vi "Create All Message Queues.vi"(8 "error in (no error)":errorcluster) -> (0 "error out":errorcluster, 3 "Message Queues out":T1)   [LabVIEW 2023, in "Tenney Message Queue.lvlib"]
doc: "This VI creates and initializes all the message queues for your application. If your application requires more than one message queue, right-click the \"Message Queues\" constant above and select Open Type Def. Add the new Message Queue(s) to the type definition, then initialize them in this VI."
uses:
  Tenney Message Queue.lvlib
  All Message Queues.ctl
  Message Cluster.ctl
  Enqueue Message (Single).vi
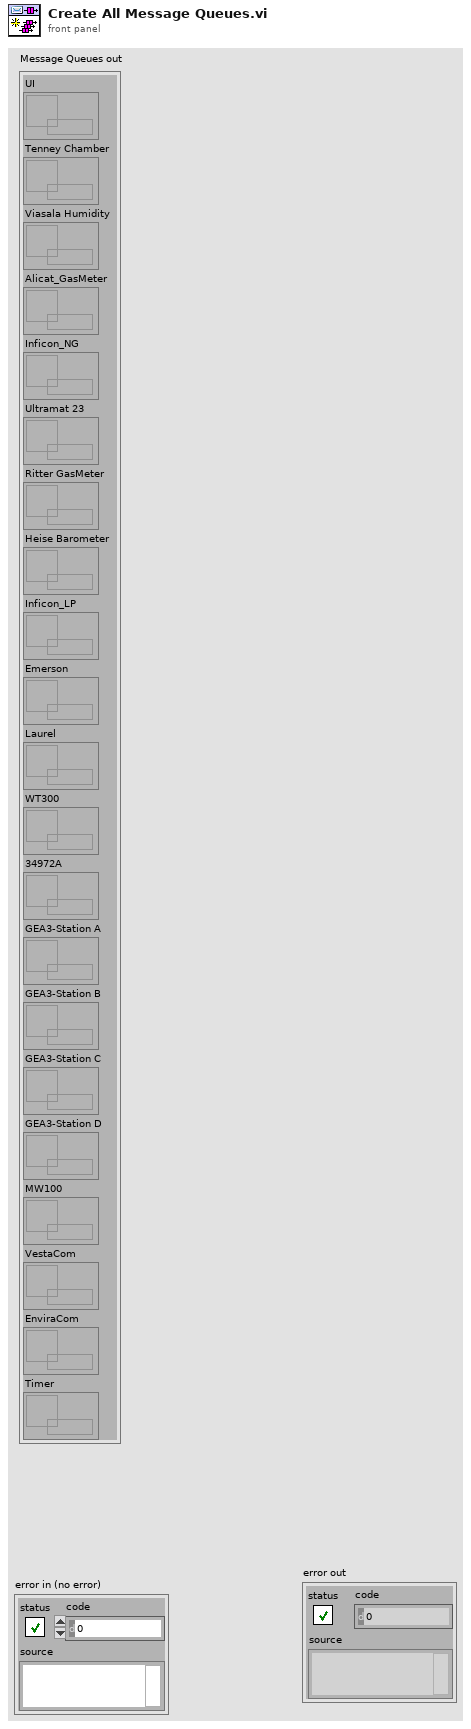
[diagram p1: front panel]
types:
  T1 = typedef "Tenney Message Queue.lvlib/All Message Queues.ctl" = cluster{"UI":refnum<queue>, "Tenney Chamber":refnum<queue>, "Viasala Humidity":refnum<queue>, "Alicat_GasMeter":refnum<queue>, "Inficon_NG":refnum<queue>, "Ultramat 23":refnum<queue>, "Ritter GasMeter":refnum<queue>, "Heise Barometer":refnum<queue>, "Inficon_LP":refnum<queue>, "Emerson":refnum<queue>, "Laurel":refnum<queue>, "WT300":refnum<queue>, "34972A":refnum<queue>, "GEA3-Station A":refnum<queue>, "GEA3-Station B":refnum<queue>, "GEA3-Station C":refnum<queue>, "GEA3-Station D":refnum<queue>, "MW100":refnum<queue>, "VestaCom":refnum<queue>, "EnviraCom":refnum<queue>, "Timer":refnum<queue>}
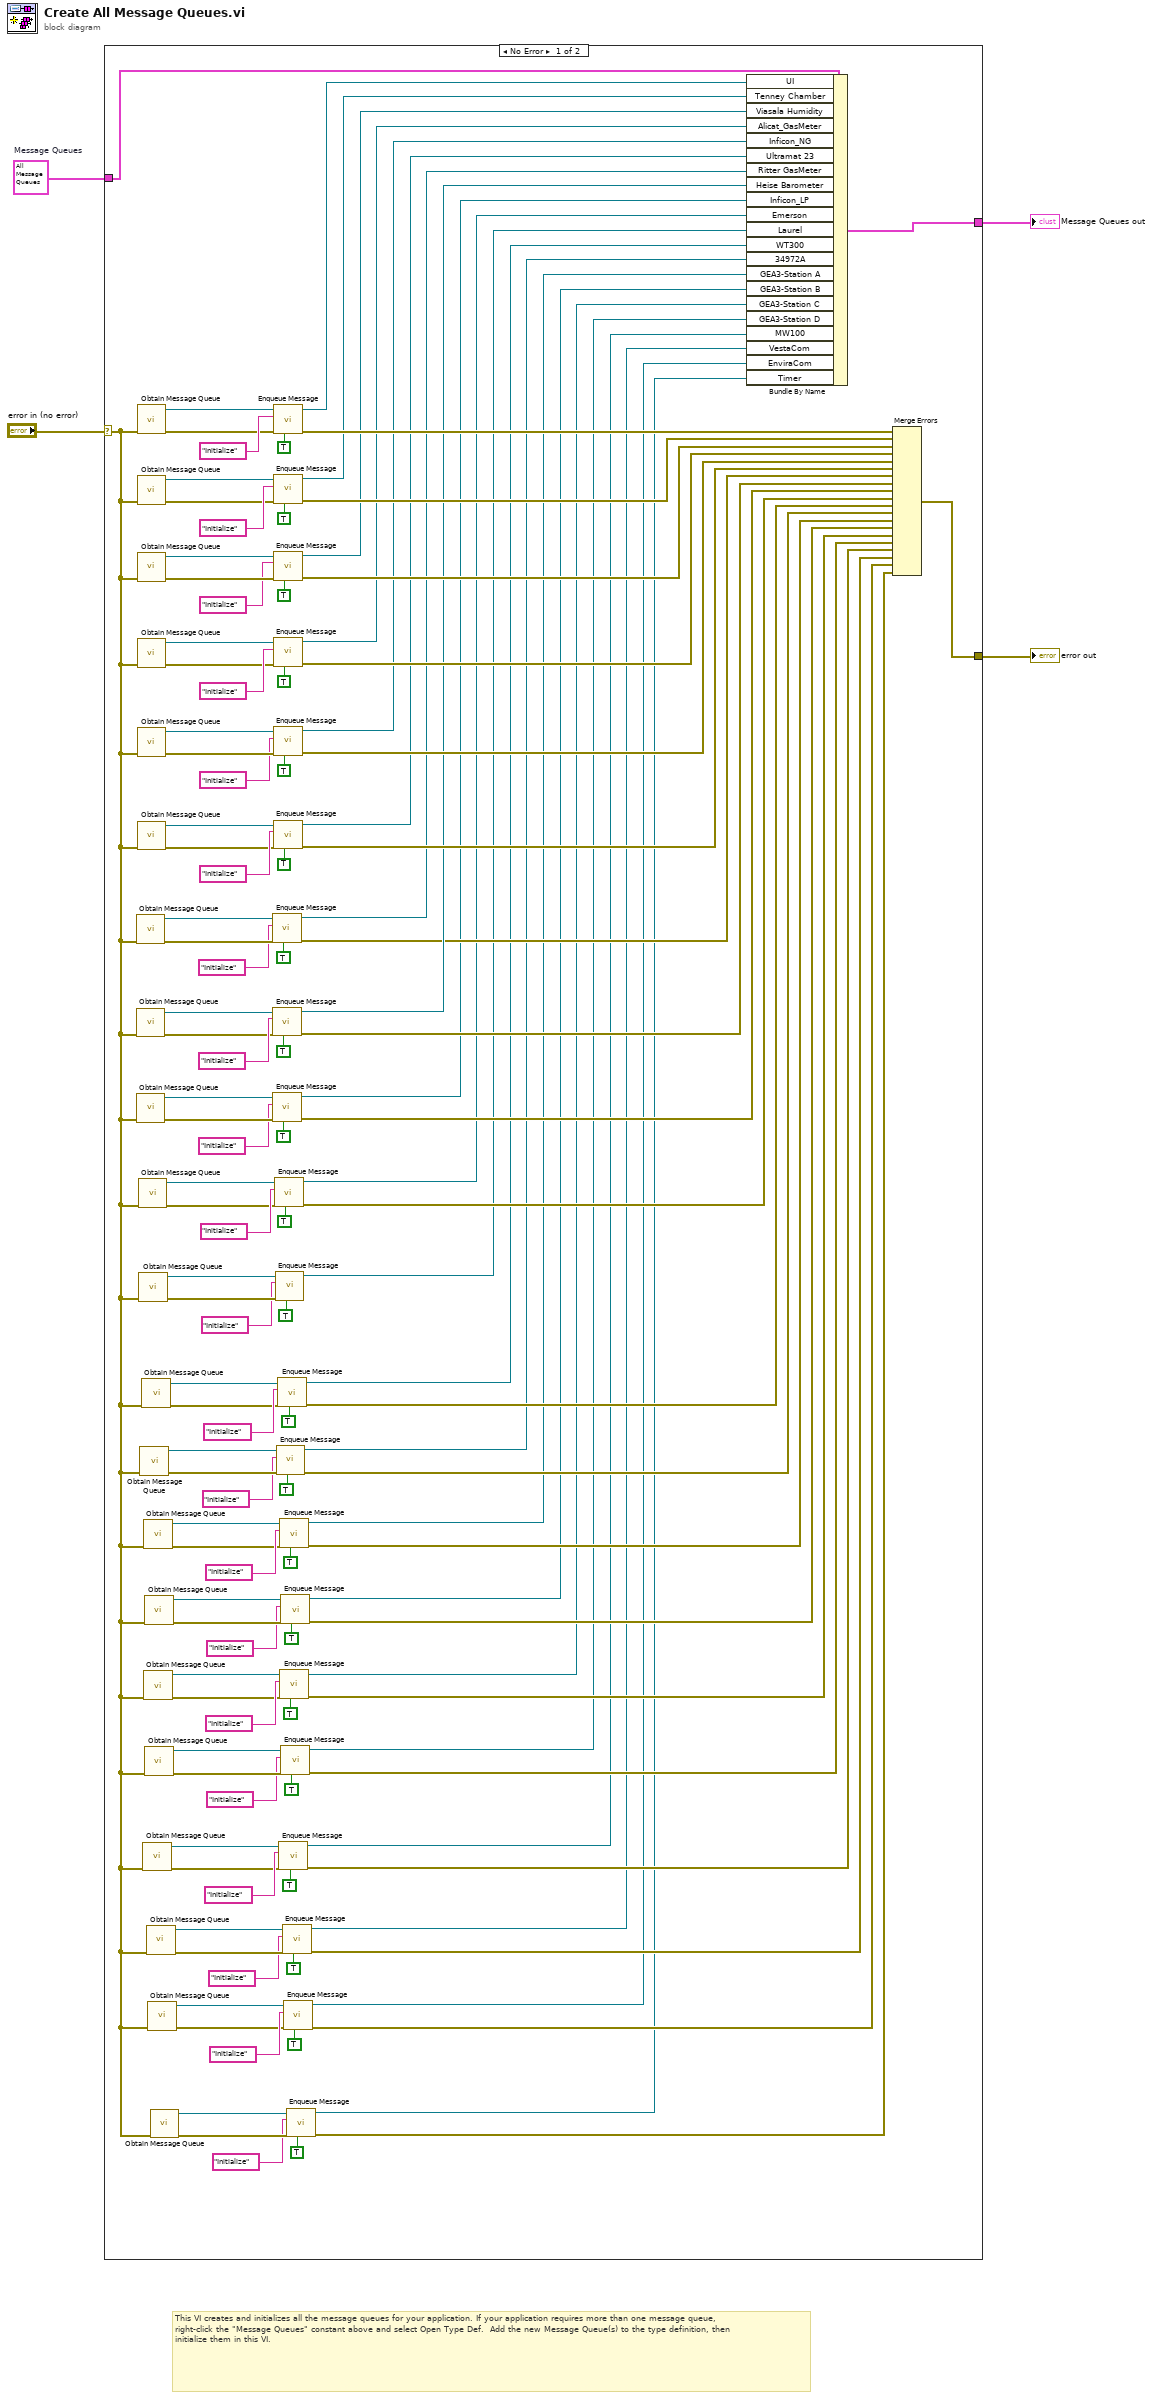
[diagram p0: block diagram]
diagram:
  w1 = T1 {"UI"=refnum, "Tenney Chamber"=refnum, "Viasala Humidity"=refnum, "Alicat_GasMeter"=refnum, "Inficon_NG"=refnum, "Ultramat 23"=refnum, "Ritter GasMeter"=refnum, "Heise Barometer"=refnum, "Inficon_LP"=refnum, "Emerson"=refnum, "Laurel"=refnum, "WT300"=refnum, "34972A"=refnum, "GEA3-Station A"=refnum, "GEA3-Station B"=refnum, "GEA3-Station C"=refnum, "GEA3-Station D"=refnum, "MW100"=refnum, "VestaCom"=refnum, "EnviraCom"=refnum, "Timer"=refnum}  # Message Queues
  # "This VI creates and initializes all the message queues for your application. If your application requires more than one message queue, right-click the \"Message Queues\" constant above and select Open Type Def.  Add the new Message Queue(s) to the type definition, then initialize them in this VI."
  n1 = case shown="No Error" "error in (no error)" {
    selector: "error in (no error)" -> [w7 w135]
    tunnel: [w127 w135] -> w4
    tunnel: [w133 w134] -> w3
    tunnel: w1 -> [w126 w134]
    frame No Error {
      n2 = call "Obtain Message Queue.vi"("error in (no error)"=w7) -> ("error out"=w94:errorcluster, "Message Queue"=w93:refnum<queue>)  [unwired: 9 in]
      n3 = call "Obtain Message Queue.vi"("error in (no error)"=w7) -> ("error out"=w87:errorcluster, "Message Queue"=w88:refnum<queue>)  [unwired: 9 in]
      n4 = call "Obtain Message Queue.vi"("error in (no error)"=w7) -> ("error out"=w82:errorcluster, "Message Queue"=w81:refnum<queue>)  [unwired: 9 in]
      n5 = call "Obtain Message Queue.vi"("error in (no error)"=w7) -> ("error out"=w130:errorcluster, "Message Queue"=w131:refnum<queue>)  [unwired: 9 in]
      n6 = call "Obtain Message Queue.vi"("error in (no error)"=w7) -> ("error out"=w119:errorcluster, "Message Queue"=w120:refnum<queue>)  [unwired: 9 in]
      n7 = call "Obtain Message Queue.vi"("error in (no error)"=w7) -> ("error out"=w118:errorcluster, "Message Queue"=w117:refnum<queue>)  [unwired: 9 in]
      n8 = call "Obtain Message Queue.vi"("error in (no error)"=w7) -> ("error out"=w109:errorcluster, "Message Queue"=w110:refnum<queue>)  [unwired: 9 in]
      n9 = call "Obtain Message Queue.vi"("error in (no error)"=w7) -> ("error out"=w106:errorcluster, "Message Queue"=w105:refnum<queue>)  [unwired: 9 in]
      n10 = call "Obtain Message Queue.vi"("error in (no error)"=w7) -> ("error out"=w97:errorcluster, "Message Queue"=w98:refnum<queue>)  [unwired: 9 in]
      n11 = call "Obtain Message Queue.vi"("error in (no error)"=w7) -> ("error out"=w73:errorcluster, "Message Queue"=w74:refnum<queue>)  [unwired: 9 in]
      n12 = call "Obtain Message Queue.vi"("error in (no error)"=w7) -> ("error out"=w70:errorcluster, "Message Queue"=w69:refnum<queue>)  [unwired: 9 in]
      n13 = call "Obtain Message Queue.vi"("error in (no error)"=w7) -> ("error out"=w59:errorcluster, "Message Queue"=w58:refnum<queue>)  [unwired: 9 in]
      n14 = call "Obtain Message Queue.vi"("error in (no error)"=w7) -> ("error out"=w62:errorcluster, "Message Queue"=w63:refnum<queue>)  [unwired: 9 in]
      n15 = call "Obtain Message Queue.vi"("error in (no error)"=w7) -> ("error out"=w26:errorcluster, "Message Queue"=w27:refnum<queue>)  [unwired: 9 in]
      n16 = call "Obtain Message Queue.vi"("error in (no error)"=w7) -> ("error out"=w50:errorcluster, "Message Queue"=w51:refnum<queue>)  [unwired: 9 in]
      n17 = call "Obtain Message Queue.vi"("error in (no error)"=w7) -> ("error out"=w42:errorcluster, "Message Queue"=w43:refnum<queue>)  [unwired: 9 in]
      n18 = call "Obtain Message Queue.vi"("error in (no error)"=w7) -> ("error out"=w49:errorcluster, "Message Queue"=w48:refnum<queue>)  [unwired: 9 in]
      n19 = call "Obtain Message Queue.vi"("error in (no error)"=w7) -> ("error out"=w41:errorcluster, "Message Queue"=w40:refnum<queue>)  [unwired: 9 in]
      n20 = call "Obtain Message Queue.vi"("error in (no error)"=w7) -> ("error out"=w23:errorcluster, "Message Queue"=w22:refnum<queue>)  [unwired: 9 in]
      n21 = call "Obtain Message Queue.vi"("error in (no error)"=w7) -> ("error out"=w16:errorcluster, "Message Queue"=w17:refnum<queue>)  [unwired: 9 in]
      n22 = call "Obtain Message Queue.vi"("error in (no error)"=w7) -> ("error out"=w11:errorcluster, "Message Queue"=w10:refnum<queue>)  [unwired: 9 in]
      n23 = call-poly "Enqueue Message.vi"("Priority Message? (F)"=TRUE, "error in (no error)"=w94, "Message"="Initialize", "Message Queue"=w93) -> ("error out"=w84:errorcluster, "dup Message Queue"=w86:refnum<queue>)  [unwired: 6 in]
      n24 = call-poly "Enqueue Message.vi"("Priority Message? (F)"=TRUE, "error in (no error)"=w87, "Message"="Initialize", "Message Queue"=w88) -> ("error out"=w83:errorcluster, "dup Message Queue"=w85:refnum<queue>)  [unwired: 6 in]
      n25 = call-poly "Enqueue Message.vi"("Priority Message? (F)"=TRUE, "error in (no error)"=w82, "Message"="Initialize", "Message Queue"=w81) -> ("error out"=w78:errorcluster, "dup Message Queue"=w77:refnum<queue>)  [unwired: 6 in]
      n26 = call-poly "Enqueue Message.vi"("Priority Message? (F)"=TRUE, "error in (no error)"=w130, "Message"="Initialize", "Message Queue"=w131) -> ("error out"=w128:errorcluster, "dup Message Queue"=w129:refnum<queue>)  [unwired: 6 in]
      n27 = call-poly "Enqueue Message.vi"("Priority Message? (F)"=TRUE, "error in (no error)"=w119, "Message"="Initialize", "Message Queue"=w120) -> ("error out"=w125:errorcluster, "dup Message Queue"=w124:refnum<queue>)  [unwired: 6 in]
      n28 = call-poly "Enqueue Message.vi"("Priority Message? (F)"=TRUE, "error in (no error)"=w118, "Message"="Initialize", "Message Queue"=w117) -> ("error out"=w114:errorcluster, "dup Message Queue"=w113:refnum<queue>)  [unwired: 6 in]
      n29 = call-poly "Enqueue Message.vi"("Priority Message? (F)"=TRUE, "error in (no error)"=w109, "Message"="Initialize", "Message Queue"=w110) -> ("error out"=w108:errorcluster, "dup Message Queue"=w107:refnum<queue>)  [unwired: 6 in]
      n30 = call-poly "Enqueue Message.vi"("Priority Message? (F)"=TRUE, "error in (no error)"=w106, "Message"="Initialize", "Message Queue"=w105) -> ("error out"=w101:errorcluster, "dup Message Queue"=w102:refnum<queue>)  [unwired: 6 in]
      n31 = call-poly "Enqueue Message.vi"("Priority Message? (F)"=TRUE, "error in (no error)"=w97, "Message"="Initialize", "Message Queue"=w98) -> ("error out"=w96:errorcluster, "dup Message Queue"=w95:refnum<queue>)  [unwired: 6 in]
      n32 = call-poly "Enqueue Message.vi"("Priority Message? (F)"=TRUE, "error in (no error)"=w73, "Message"="Initialize", "Message Queue"=w74) -> ("error out"=w72:errorcluster, "dup Message Queue"=w71:refnum<queue>)  [unwired: 6 in]
      n33 = call-poly "Enqueue Message.vi"("Priority Message? (F)"=TRUE, "error in (no error)"=w70, "Message"="Initialize", "Message Queue"=w69) -> ("dup Message Queue"=w66:refnum<queue>)  [unwired: 6 in, 1 out]
      n34 = call-poly "Enqueue Message.vi"("Priority Message? (F)"=TRUE, "error in (no error)"=w59, "Message"="Initialize", "Message Queue"=w58) -> ("error out"=w55:errorcluster, "dup Message Queue"=w54:refnum<queue>)  [unwired: 6 in]
      n35 = call-poly "Enqueue Message.vi"("Priority Message? (F)"=TRUE, "error in (no error)"=w62, "Message"="Initialize", "Message Queue"=w63) -> ("error out"=w60:errorcluster, "dup Message Queue"=w61:refnum<queue>)  [unwired: 6 in]
      n36 = call-poly "Enqueue Message.vi"("Priority Message? (F)"=TRUE, "error in (no error)"=w26, "Message"="Initialize", "Message Queue"=w27) -> ("error out"=w25:errorcluster, "dup Message Queue"=w24:refnum<queue>)  [unwired: 6 in]
      n37 = call-poly "Enqueue Message.vi"("Priority Message? (F)"=TRUE, "error in (no error)"=w50, "Message"="Initialize", "Message Queue"=w51) -> ("error out"=w37:errorcluster, "dup Message Queue"=w33:refnum<queue>)  [unwired: 6 in]
      n38 = call-poly "Enqueue Message.vi"("Priority Message? (F)"=TRUE, "error in (no error)"=w42, "Message"="Initialize", "Message Queue"=w43) -> ("error out"=w35:errorcluster, "dup Message Queue"=w31:refnum<queue>)  [unwired: 6 in]
      n39 = call-poly "Enqueue Message.vi"("Priority Message? (F)"=TRUE, "error in (no error)"=w49, "Message"="Initialize", "Message Queue"=w48) -> ("error out"=w36:errorcluster, "dup Message Queue"=w32:refnum<queue>)  [unwired: 6 in]
      n40 = call-poly "Enqueue Message.vi"("Priority Message? (F)"=TRUE, "error in (no error)"=w41, "Message"="Initialize", "Message Queue"=w40) -> ("error out"=w34:errorcluster, "dup Message Queue"=w30:refnum<queue>)  [unwired: 6 in]
      n41 = call-poly "Enqueue Message.vi"("Priority Message? (F)"=TRUE, "error in (no error)"=w23, "Message"="Initialize", "Message Queue"=w22) -> ("error out"=w15:errorcluster, "dup Message Queue"=w13:refnum<queue>)  [unwired: 6 in]
      n42 = call-poly "Enqueue Message.vi"("Priority Message? (F)"=TRUE, "error in (no error)"=w16, "Message"="Initialize", "Message Queue"=w17) -> ("error out"=w14:errorcluster, "dup Message Queue"=w12:refnum<queue>)  [unwired: 6 in]
      n43 = call-poly "Enqueue Message.vi"("Priority Message? (F)"=TRUE, "error in (no error)"=w11, "Message"="Initialize", "Message Queue"=w10) -> ("error out"=w6:errorcluster, "dup Message Queue"=w5:refnum<queue>)  [unwired: 6 in]
      n44 = Bundle By Name(cluster=w126, "UI"=w129, "Tenney Chamber"=w124, "Viasala Humidity"=w113, "Alicat_GasMeter"=w107, "Inficon_NG"=w102, "Ultramat 23"=w95, "Ritter GasMeter"=w86, "Heise Barometer"=w85, "Inficon_LP"=w77, "Emerson"=w71, "Laurel"=w66, "WT300"=w61, "34972A"=w54, "GEA3-Station A"=w33, "GEA3-Station B"=w32, "GEA3-Station C"=w31, "GEA3-Station D"=w30, "MW100"=w24, "VestaCom"=w13, "EnviraCom"=w12, "Timer"=w5) -> (w133:T1)
      n45 = Merge Errors(w128, w125, w114, w108, w101, w96, w84, w83, w78, w72, w60, w55, w37, w36, w35, w34, w25, w15, w14, w6) -> (w127:errorcluster)
    }
    frame Error {
    }
  }
  "Message Queues out" <- w3
  "error out" <- w4
